vi "Test two motor readings.vi"() -> ()   [LabVIEW 2016]
uses:
  <vilib>/Platform/TimedLoop/XDataNode/timing_clust.ctl
  <vilib>/Platform/TimedLoop/XDataNode/nitl_modes.ctl
  <vilib>/Platform/TimedLoop/XDataNode/wakeup.ctl
  Motor controllers.vi
  <vilib>/CANopenLib/CANOPEN.llb/CANopen SDO Create.vi
  Set into drive mode.vi
  <vilib>/CANopenLib/CANOPEN.llb/CANopen SDO Close.vi
  Get Actual Position.vi
  <vilib>/Platform/TimedLoop/XDataNode/XDataNode.xnode
  <vilib>/Platform/TimedLoop/XDataNode/XDNodeRunTimeDep.lvlib
panel:
  out "error out":errorcluster
  out "Waveform Chart":cluster{"I32 data":i32, "I32 data":i32}(graph)
  in  "Stop Button":bool
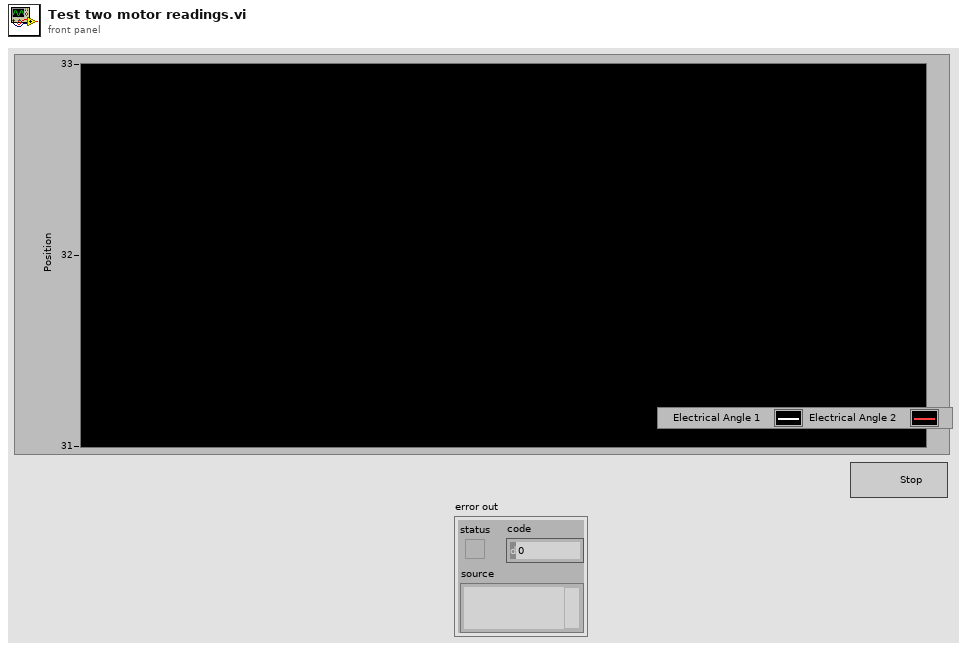
[diagram p1: front panel]
types:
  T1 = typedef "XDNodeRunTimeDep.lvlib/timing_clust.ctl" = cluster{"Expected End [f-1]":u64, "Actual End [f-1]":u64, "Finished Late? [f-1]":bool, "Expected End [i-1]":u64, "Actual End [i-1]":u64, "Finished Late? [i-1]":bool, "Expected Start [i]":u64, "Actual Start [i]":u64, "Expected Start [f]":u64, "Actual Start [f]":u64, "Source Name":string, "Structure Name":string, "Period":i64, "Deadline":i64, "Offset":i64, "Start":i64, "Priority":i32, "Timeout":i32, "Mode":T2, "Wakeup Reason":T3, "Error":errorcluster, "Source Type":string, "Secondary Source Type":string, "Global End Time":u64, "Global Start Time":u64, "Frame Duration":u64, "Iteration Duration":u64, "Assigned CPU":i32, "I/O Scan Engine Mode":u32}
  T2 = typedef "XDNodeRunTimeDep.lvlib/nitl_modes.ctl" = enum32{"No Change", "Process missed periods, maintain original phase", "Discard missed periods, maintain original phase", "Process missed periods, ignore original phase", "Discard missed periods, ignore original phase"}
  T3 = typedef "XDNodeRunTimeDep.lvlib/wakeup.ctl" = enum32{"Normal", "Aborted", "Asynchronous wakeup", "Timing source error", "Timed loop error", "Timeout"}
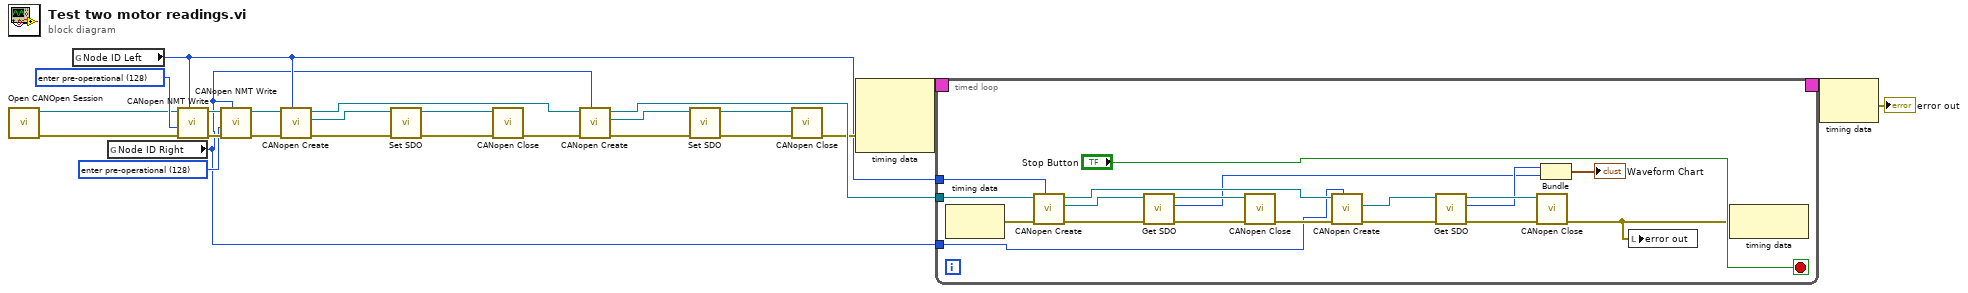
[diagram p0: block diagram]
diagram:
  w21 = u16 128 items=["start remote node"=1, "stop remote node"=2, "enter pre-operational"=128, "reset node"=129, "reset communication"=130] ("command")
  w22 = u16 128 items=["start remote node"=1, "stop remote node"=2, "enter pre-operational"=128, "reset node"=129, "reset communication"=130] ("command")
  n1 = call "Open CANOpen Session.vi"() -> ("error out"=w19:errorcluster, "interface object out"=w18:refnum<k20>)  [unwired: 10 in]
  n2 = global read "Motor controllers.vi" "Node ID Left"() -> (w2:u8)
  n3 = global read "Motor controllers.vi" "Node ID Right"() -> (w1:u8)
  n4 = call <vilib>:"CANopen NMT Write.vi"("node-ID (0)"=w2, "error in (no error)"=w19, "command"=w22, "interface object in"=w18) -> ("error out"=w23:errorcluster, "interface object out"=w20:refnum<k20>)  [unwired: 6 in]
  n5 = call <vilib>:"CANopen NMT Write.vi"("node-ID (0)"=w1, "error in (no error)"=w23, "command"=w21, "interface object in"=w20) -> ("error out"=w4:errorcluster, "interface object out"=w6:refnum<k20>)  [unwired: 6 in]
  n6 = call-poly <vilib>:"CANopen Create.vi"("node-ID"=w2, "error in (no error)"=w4, "interface object in"=w6) -> ("error out"=w13:errorcluster, "SDO object out"=w16:refnum<k20>, "interface object out"=w8:refnum<k20>)  [unwired: 6 in]
  n7 = call-poly "Set SDO.vi"("error in (no error)"=w13, "SDO object in"=w16) -> ("error out"=w14:errorcluster, "SDO object out"=w15:refnum<k20>)  [unwired: 8 in]
  n8 = call-poly <vilib>:"CANopen Close.vi"("error in (no error)"=w14, "SDO object in"=w15) -> ("error out"=w7:errorcluster)  [unwired: 9 in]
  n9 = call-poly <vilib>:"CANopen Create.vi"("node-ID"=w1, "error in (no error)"=w7, "interface object in"=w8) -> ("error out"=w9:errorcluster, "SDO object out"=w12:refnum<k20>, "interface object out"=w5:refnum<k20>)  [unwired: 6 in]
  n10 = call-poly "Set SDO.vi"("error in (no error)"=w9, "SDO object in"=w12) -> ("error out"=w10:errorcluster, "SDO object out"=w11:refnum<k20>)  [unwired: 8 in]
  n11 = call-poly <vilib>:"CANopen Close.vi"("error in (no error)"=w10, "SDO object in"=w11) -> ("error out"=w3:errorcluster)  [unwired: 9 in]
  n12 = node-c288(w3) -> (w25:T1)  [unwired: 2 in]
  n13 = timed-loop {
    timing: w25 -> [_]
    timing-out: [_] -> w24
    tunnel: w5 -> [w40]
    tunnel: w2 -> [w30]
    tunnel: w1 -> [w29]
    stop <- "Stop Button" stop-if-true
    n14 = node-c288() -> (w41:errorcluster)  [unwired: 1 in]
    n15 = call-poly <vilib>:"CANopen Create.vi"("node-ID"=w30, "error in (no error)"=w41, "interface object in"=w40) -> ("error out"=w42:errorcluster, "SDO object out"=w39:refnum<k20>, "interface object out"=w36:refnum<k20>)  [unwired: 6 in]
    n16 = call-poly "Get SDO.vi"("error in (no error)"=w42, "SDO object in"=w39) -> ("error out"=w34:errorcluster, "I32 data"=w27:i32, "SDO object out"=w35:refnum<k20>)  [unwired: 6 in, 1 out]
    n17 = call-poly <vilib>:"CANopen Close.vi"("error in (no error)"=w34, "SDO object in"=w35) -> ("error out"=w33:errorcluster)  [unwired: 9 in]
    n18 = call-poly <vilib>:"CANopen Create.vi"("node-ID"=w29, "error in (no error)"=w33, "interface object in"=w36) -> ("error out"=w37:errorcluster, "SDO object out"=w38:refnum<k20>)  [unwired: 6 in, 1 out]
    n19 = call-poly "Get SDO.vi"("error in (no error)"=w37, "SDO object in"=w38) -> ("error out"=w31:errorcluster, "I32 data"=w28:i32, "SDO object out"=w32:refnum<k20>)  [unwired: 6 in, 1 out]
    n20 = call-poly <vilib>:"CANopen Close.vi"("error in (no error)"=w31, "SDO object in"=w32) -> ("error out"=w26:errorcluster)  [unwired: 9 in]
    n21 = Bundle("I32 data"=w28, "I32 data"=w27) -> (→"Waveform Chart":cluster{"I32 data":i32, "I32 data":i32})  [unwired: 1 in]
    n22 = local write "error out"(w26) -> ()
    n23 = node-c288(w26) -> ()  [unwired: 1 out]
  }
  n24 = node-c288(w24) -> (→"error out":errorcluster)
